vi "buffer array 2D.vi"(0 "Array":i32[][](array[numeric]), 1 "History length":i32, 2 "Log":T1=enum."TimeStamp", 10 "Start channel":i32) -> (14 "Vmon History":i32[][][](array[numeric]))   [LabVIEW 2018]
uses:
  history_array_type.ctl
panel:
  out "channel history":i32[][](array[numeric])
  in  "channel":i32
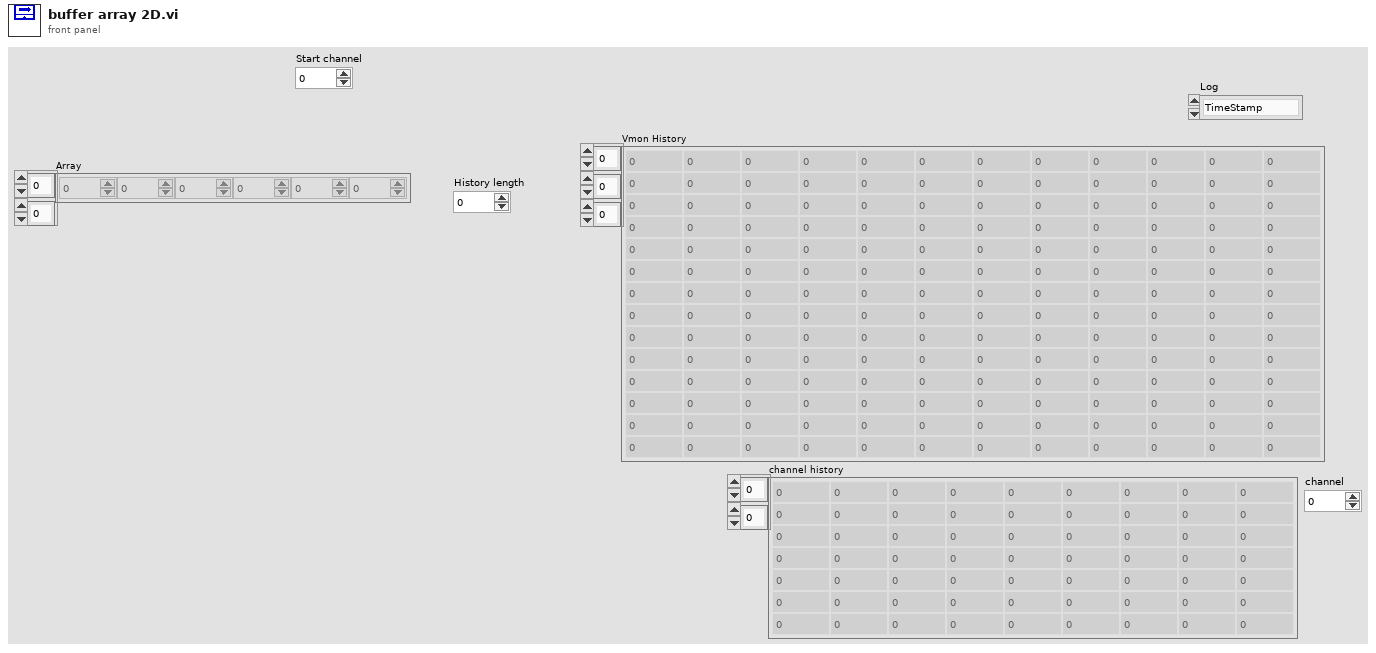
[diagram p1: front panel]
types:
  T1 = typedef "history_array_type.ctl" = enum16{"Vmon", "Vset", "Imon", "Iset", "TimeStamp"}
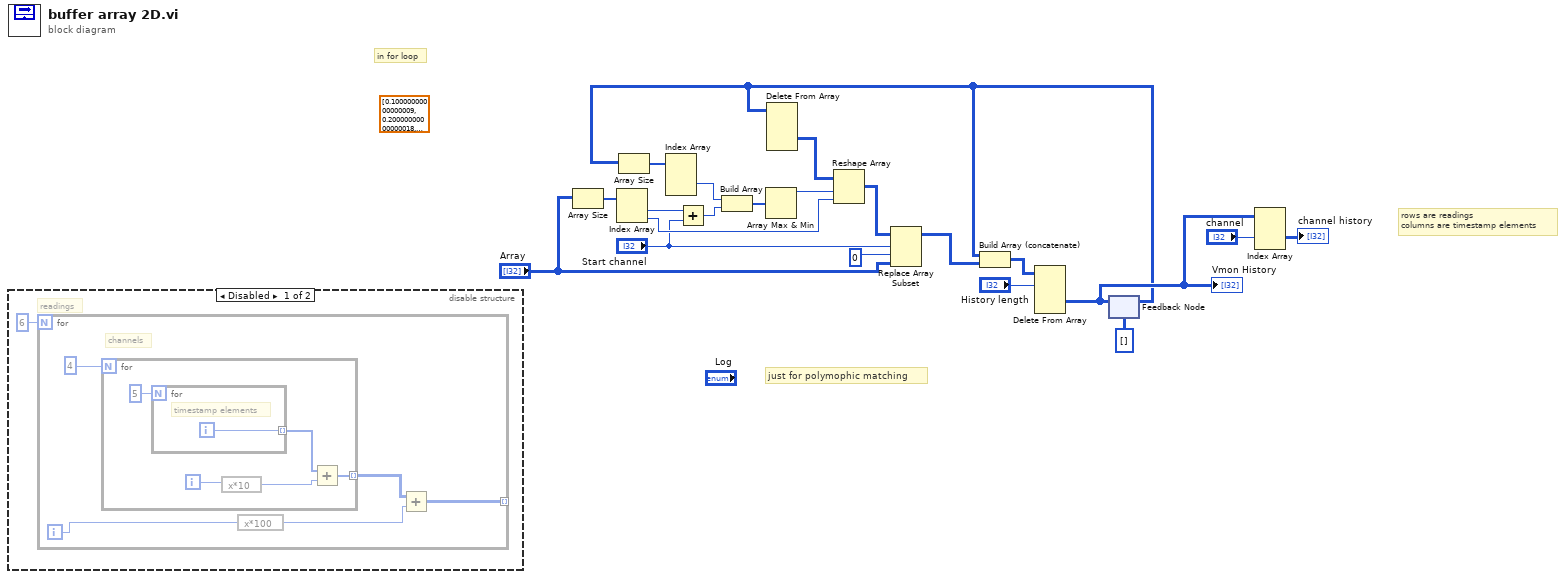
[diagram p0: block diagram]
diagram:
  (unwired) dbl[][] [[0.10000000000000009, 0.20000000000000018, 1.2999999999999998], [1.1, 1.2, 1.3], [2.1, 2.2, 2.3], [3.1, 3.2, 3.3], [4.1, 4.2, 4.3], [5.1, 5.2, 5.3]] ("Test")
  # "just for polymophic matching"
  # "rows are readings\ncolumns are timestamp elements"
  # "in for loop"
  n1 = disable-structure shown="Disabled" {
    frame Disabled {
      # "readings"
      n2 = for {
        N: 6 -> [_]
        tunnel: [w23] -> _ mode=indexing
        i -> [w26]
        # "channels"
        n3 = for {
          N: 4 -> [_]
          tunnel: [w28] -> w25 mode=indexing
          i -> [w31]
          n4 = for {
            N: 5 -> [_]
            tunnel: [w33] -> w30 mode=indexing
            i -> [w33]
            # "timestamp elements"
          }
          n5 = expression code="x*10"(w31) -> (w29:i32)
          n6 = Add(x=w30, y=w29) -> (x+y=w28:i32[])
        }
        n7 = expression code="x*100"(w26) -> (w24:i32)
        n8 = Add(x=w25, y=w24) -> (x+y=w23:i32[][])
      }
    }
    frame Enabled {
    }
  }
  n9 = Array Size(array="Array") -> (size(s)=w13:i32[])
  n10 = Index Array(array=w13) -> (element #1=w12:i32, element #2=w4:i32)  [unwired: 2 in]
  n11 = Add(x=w12, y="Start channel") -> (x+y=w11:i32)
  n12 = feedback #1(i32[][][] [] ("Vmon History")) -> (w8:i32[][][])
  n13 = Array Size(array=w8) -> (size(s)=w14:i32[])
  n14 = Index Array(array=w14) -> (element #2=w1:i32)  [unwired: 3 in, 2 out]
  n15 = Build Array(w1, w11) -> (w15:i32[])
  n16 = Array Max & Min(array=w15) -> (max value=w5:i32)  [unwired: 3 out]
  n17 = Delete From Array(array=w8) -> (deleted portion=w10:i32[][])  [unwired: 4 in, 1 out]
  n18 = Reshape Array(w10, w5, w4) -> (w9:i32[][])
  n19 = Replace Array Subset(array=w9, new element="Array", index (row)="Start channel", index (col)=0 ("disabled index (row)")) -> (w7:i32[][])
  n20 = Build Array (concatenate)(w8, w7) -> (w17:i32[][][])
  n21 = Delete From Array(array=w17, length="History length") -> (deleted portion=w21:i32[][][])  [unwired: 3 in, 1 out]
  "Vmon History" <- w21
  n22 = feedback-in #1(w21) -> ()
  n23 = Index Array(array=w21, index (dim 1)="channel") -> (element=→"channel history":i32[][])  [unwired: 2 in]
